vi "ModifyAttribute1.vi"(0 "reference in":refnum<class "G#SubClass2.lvclass">, 1 "Lock time (ms)":u32, 2 "timeout in ms (-1)":i32=-1, 3 "Unlock data if error? (T)":bool=TRUE, 4 "Only unlock data? (F)":bool, 5 "error in (no error)":errorcluster, 7 "status":bool) -> (14 "reference out":refnum<class "G#SubClass2.lvclass">, 16 "timeout":bool, 19 "error out":errorcluster)   [LabVIEW 2020, in "G#SubClass2.lvclass"]
uses:
  G#SubClass2.lvclass
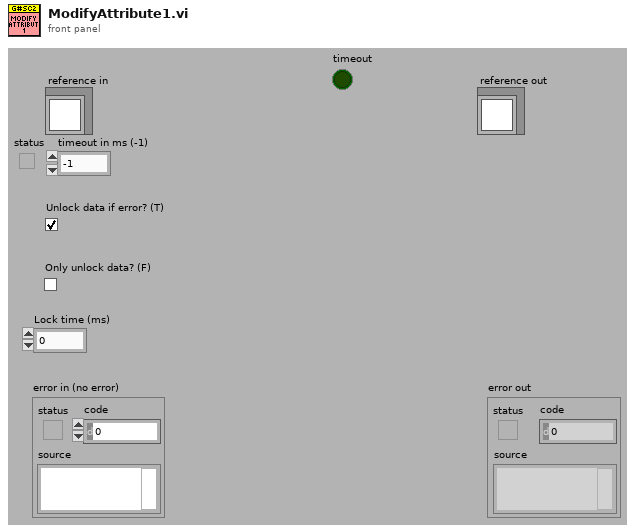
[diagram p1: front panel]
types:
  T1 = typedef "G#SubClass2.lvclass/ObjectAttributes.ctl" = cluster{"Base class":T2, "SubAttribute":dbl}
  T2 = typedef "G#BaseClass2.lvclass/ObjectAttributes.ctl" = cluster{"Numeric":dbl, "Array":dbl[]}
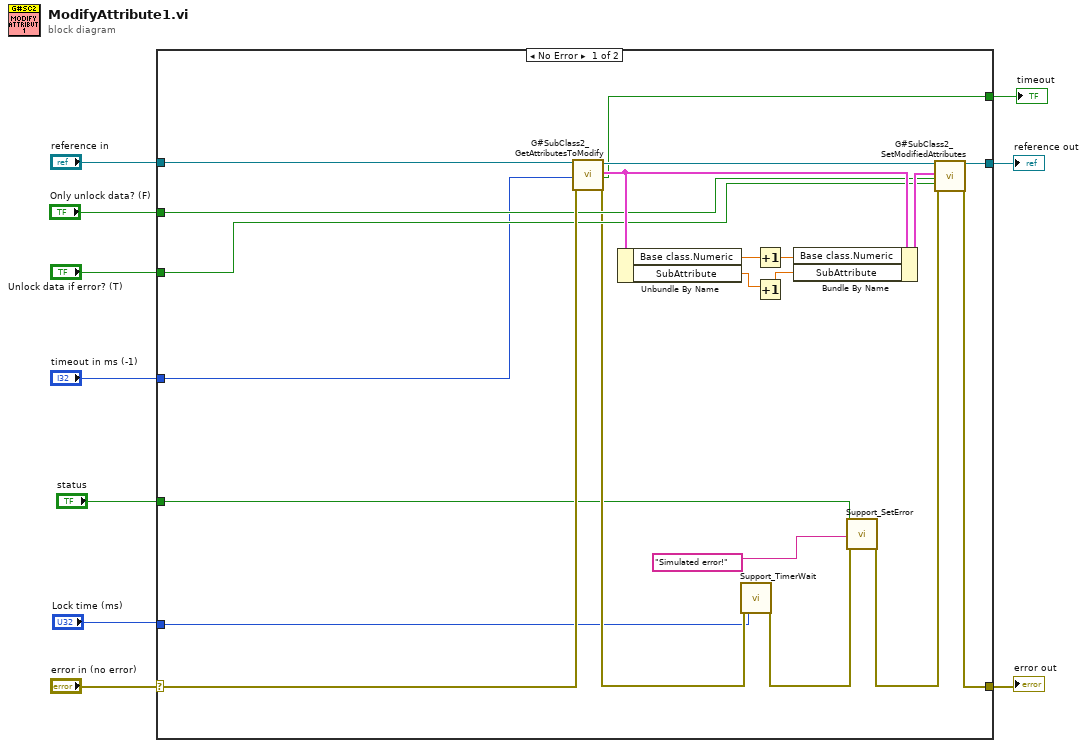
[diagram p0: block diagram]
diagram:
  n1 = case shown="No Error" "error in (no error)" {
    selector: "error in (no error)" -> [w27 w33]
    tunnel: [w29 w33] -> w9
    tunnel: [w26 w32] -> w7
    tunnel: "reference in" -> [w28 w32]
    tunnel: "Only unlock data? (F)" -> [w20 _]
    tunnel: "Unlock data if error? (T)" -> [w19 _]
    tunnel: "Lock time (ms)" -> [w17 _]
    tunnel: "status" -> [w13 _]
    tunnel: [w12 _] -> w2
    tunnel: "timeout in ms (-1)" -> [w11 _]
    frame No Error {
      n2 = call "G#SubClass2_GetAttributesToModify.vi"("reference in"=w28, "timeout in ms (-1)"=w11, "error in (no error)"=w27) -> ("reference out"=w30:refnum<class "G#SubClass2.lvclass">, "attributes"=w25:T1, "timeout"=w12:bool, "error out"=w18:errorcluster)  [unwired: 12 in, 1 out]
      n3 = Unbundle By Name(w25) -> ("Base class.Numeric"=w24:dbl, "SubAttribute"=w21:dbl)
      n4 = call "Support_TimerWait.vi"("error in (no error)"=w18, "milliseconds to wait"=w17) -> ("error out"=w16:errorcluster)  [unwired: 17 in]
      n5 = Increment(x=w24) -> (x+1=w23:dbl)
      n6 = Increment(x=w21) -> (x+1=w22:dbl)
      n7 = Bundle By Name(cluster=w25, "Base class.Numeric"=w23, "SubAttribute"=w22) -> (w31:T1)
      n8 = call "Support_SetError.vi"("status"=w13, "source"="Simulated error!", "error in (no error)"=w16) -> ("error out"=w15:errorcluster)  [unwired: 16 in]
      n9 = call "G#SubClass2_SetModifiedAttributes.vi"("reference in"=w30, "attributes"=w31, "Only unlock data? (F)"=w20, "Unlock data if error? (T)"=w19, "error in (no error)"=w15) -> ("reference out"=w26:refnum<class "G#SubClass2.lvclass">, "error out"=w29:errorcluster)  [unwired: 13 in]
    }
    frame Error {
    }
  }
  "error out" <- w9
  "reference out" <- w7
  "timeout" <- w2
